vi "homework - pico pwm with adc continuous.vi"() -> ()   [LabVIEW 2024]
doc: "#vi_description \nGenerate a PWM signal, capture on two ADCs, and plot points continuously onto a waveform chart until the user presses stop or an error has occurred.\nThetic Engineering Ltd."
uses:
  <vilib>/CTI/CTI Visa Drivers/CTI-Visa/CTI-Visa.lvlib
panel:
  out "Actual Frequency":sgl
  out "Actual Duty Cycle":sgl
  in  "Frequency":sgl(slide)=10.0 caption="Requested Frequency (10 - 100) Hz" min=0 max=10000 step=10 scale=10.0..100.0
  in  "Duty Cycle":sgl(slide)=0.5 caption="Requested Duty Cycle (0 - 1) %" min=0 max=1 step=0.1 scale=0.0..1.0
  in  "Stop":bool
  out "Waveform Chart":cluster{"Value":u16, "Value":u16}(graph)
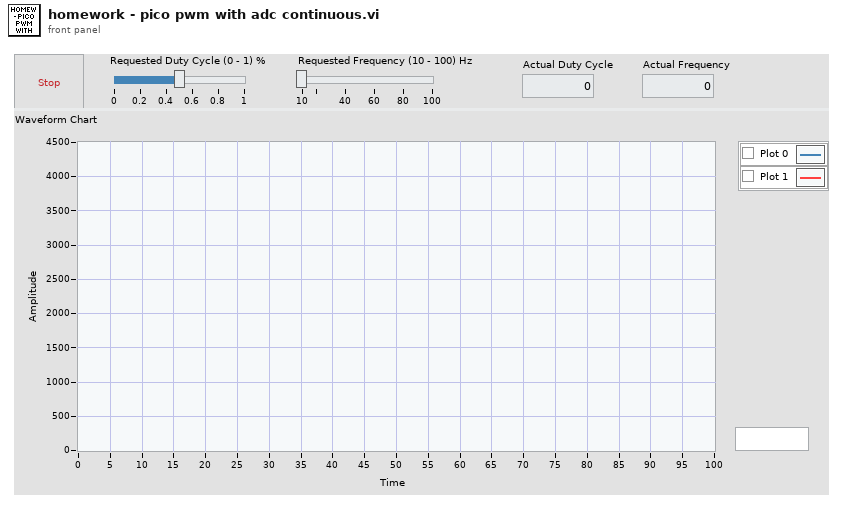
[diagram p1: front panel]
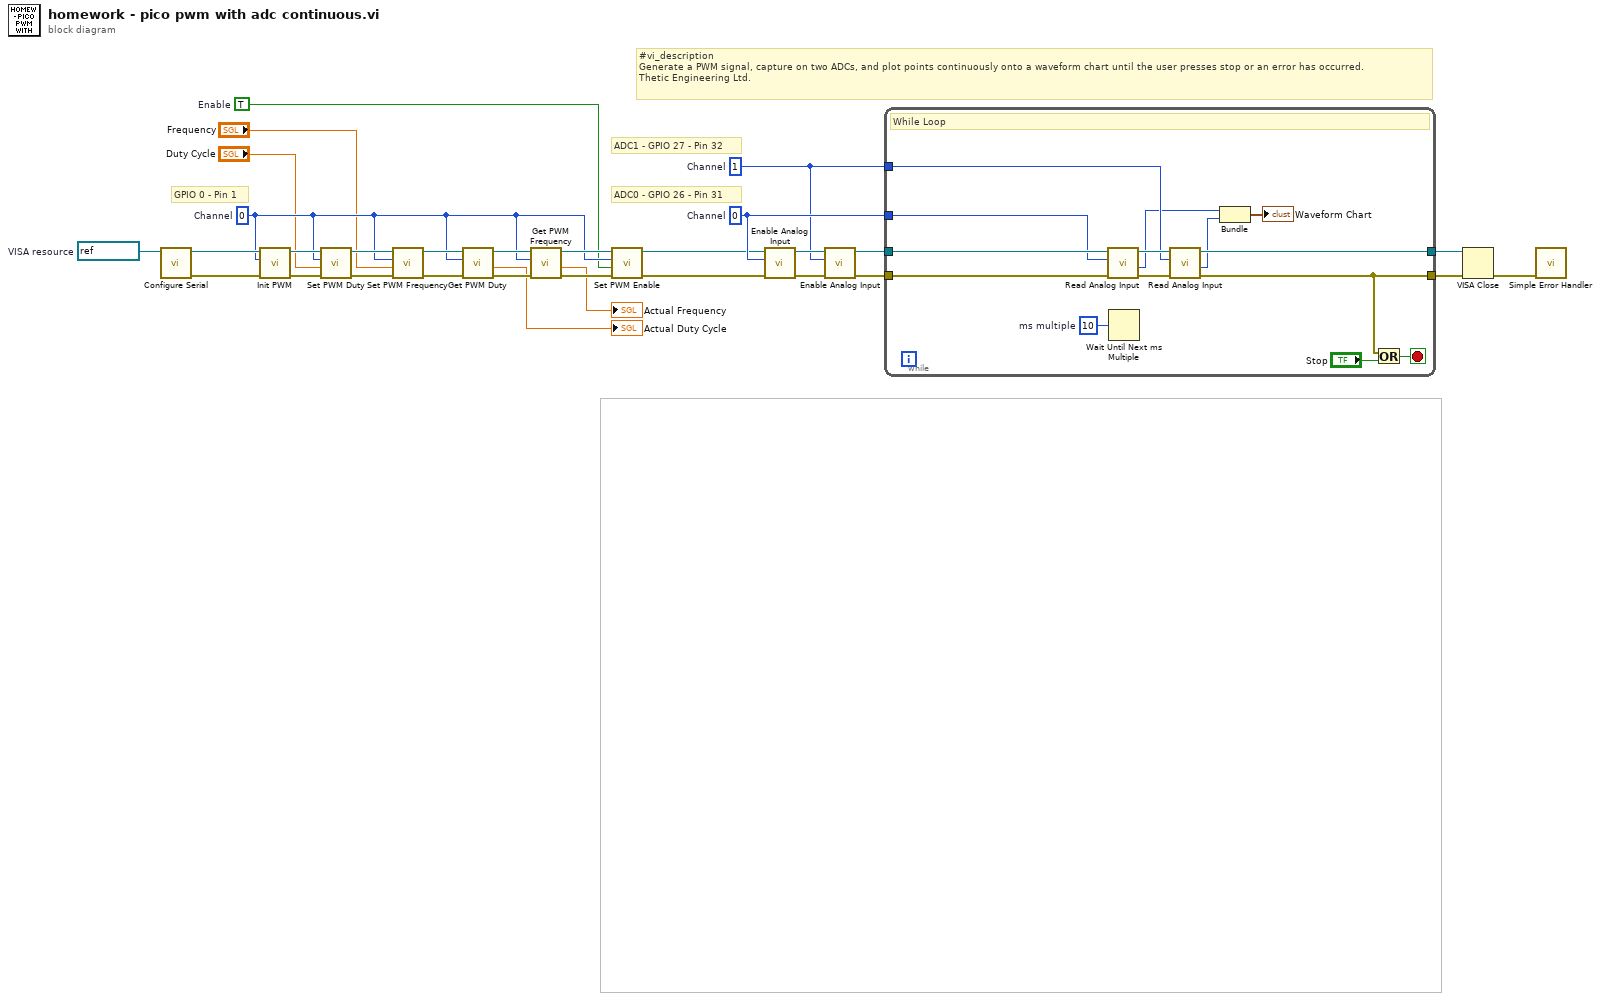
[diagram p0: block diagram]
diagram:
  w1 = TRUE  # Enable
  w6 = 0  # Channel
  w21 = 1  # Channel
  w25 = 0  # Channel
  w28 = refnum<visa-resource-name> "COM3"  # VISA resource
  # "GPIO 0 - Pin 1"
  # "ADC1 - GPIO 27 - Pin 32"
  # "ADC0 - GPIO 26 - Pin 31"
  # "#vi_description \nGenerate a PWM signal, capture on two ADCs, and plot points continuously onto a waveform chart until the user presses stop or an error has occurred.\nThetic Engineering Ltd."
  n1 = call <vilib>:"Configure Serial.vi"("VISA resource name in"=w28) -> ("error out"=w9:errorcluster, "VISA resource name"=w10:refnum<visa-resource-name>)  [unwired: 9 in]
  n2 = call <vilib>:"Init PWM.vi"("error in (no error)"=w9, "Channel"=w6, "VISA resource name in"=w10) -> ("error out"=w20:errorcluster, "VISA resource name"=w19:refnum<visa-resource-name>)  [unwired: 7 in]
  n3 = call <vilib>:"Set PWM Duty.vi"("error in (no error)"=w20, "Duty % (0-1)"="Duty Cycle", "Channel"=w6, "VISA resource name in"=w19) -> ("error out"=w17:errorcluster, "VISA resource name"=w18:refnum<visa-resource-name>)  [unwired: 6 in]
  n4 = call <vilib>:"Set PWM Frequency.vi"("error in (no error)"=w17, "Freq Hz"="Frequency", "Channel"=w6, "VISA resource name in"=w18) -> ("error out"=w15:errorcluster, "VISA resource name"=w16:refnum<visa-resource-name>)  [unwired: 6 in]
  n5 = call <vilib>:"Get PWM Duty.vi"("error in (no error)"=w15, "Channel"=w6, "VISA resource name in"=w16) -> ("error out"=w13:errorcluster, "Duty % (0-1)"=→"Actual Duty Cycle":sgl, "VISA resource name"=w14:refnum<visa-resource-name>)  [unwired: 6 in]
  n6 = call <vilib>:"Get PWM Frequency.vi"("error in (no error)"=w13, "Channel"=w6, "VISA resource name in"=w14) -> ("error out"=w11:errorcluster, "Freq Hz"=→"Actual Frequency":sgl, "VISA resource name"=w12:refnum<visa-resource-name>)  [unwired: 6 in]
  n7 = call <vilib>:"Set PWM Enable.vi"("error in (no error)"=w11, "Enable"=w1, "Channel"=w6, "VISA resource name in"=w12) -> ("error out"=w7:errorcluster, "VISA resource name"=w8:refnum<visa-resource-name>)  [unwired: 6 in]
  n8 = call <vilib>:"Enable Analog Input.vi"("error in (no error)"=w7, "Channel"=w25, "VISA resource name in"=w8) -> ("error out"=w26:errorcluster, "VISA resource name"=w23:refnum<visa-resource-name>)  [unwired: 7 in]
  n9 = call <vilib>:"Enable Analog Input.vi"("error in (no error)"=w26, "Channel"=w21, "VISA resource name in"=w23) -> ("error out"=w24:errorcluster, "VISA resource name"=w22:refnum<visa-resource-name>)  [unwired: 7 in]
  n10 = while {
    tunnel: w22 -> [w42]
    tunnel: w24 -> [w41]
    tunnel: [w35] -> w30
    tunnel: [w37] -> w29
    tunnel: w25 -> [w38]
    tunnel: w21 -> [w34]
    stop <- w40 stop-if-true
    w43 = u32 10  # ms multiple
    # "While Loop"
    n11 = call <vilib>:"Read Analog Input.vi"("error in (no error)"=w41, "Channel"=w38, "VISA resource name in"=w42) -> ("error out"=w39:errorcluster, "Value"=w32:u16, "VISA resource name"=w36:refnum<visa-resource-name>)  [unwired: 6 in]
    n12 = Wait Until Next ms Multiple(millisecond multiple=w43) -> ()  [unwired: 1 out]
    n13 = call <vilib>:"Read Analog Input.vi"("error in (no error)"=w39, "Channel"=w34, "VISA resource name in"=w36) -> ("error out"=w37:errorcluster, "Value"=w31:u16, "VISA resource name"=w35:refnum<visa-resource-name>)  [unwired: 6 in]
    n14 = Bundle("Value"=w32, "Value"=w31) -> (→"Waveform Chart":cluster{"Value":u16, "Value":u16})  [unwired: 1 in]
    n15 = Or(x=w37, y="Stop") -> (x .or. y?=w40:bool)
  }
  n16 = VISA Close(VISA resource name=w30, error in (no error)=w29) -> (error out=w27:errorcluster)
  n17 = call <vilib>:"Simple Error Handler.vi"("error in (no error)"=w27) -> ()  [unwired: 4 in, 5 out]
